vi "Event Handle Loop_Insert.vi"(8 "error in (no error)":errorcluster, 10 "Label":string, 11 "QTab Class in":refnum<class "QTab Class.lvclass">) -> (0 "error out":errorcluster, 3 "QTab Class out":refnum<class "QTab Class.lvclass">)   [LabVIEW 2020, in "QTab.lvlib" / "QTab Class.lvclass"]
uses:
  QTab Class.lvclass
  QTab Class.lvclass/QTab Class.ctl
  QMenu Class/Button Attribute.ctl
  QMenu Class/QMenu Class.lvclass
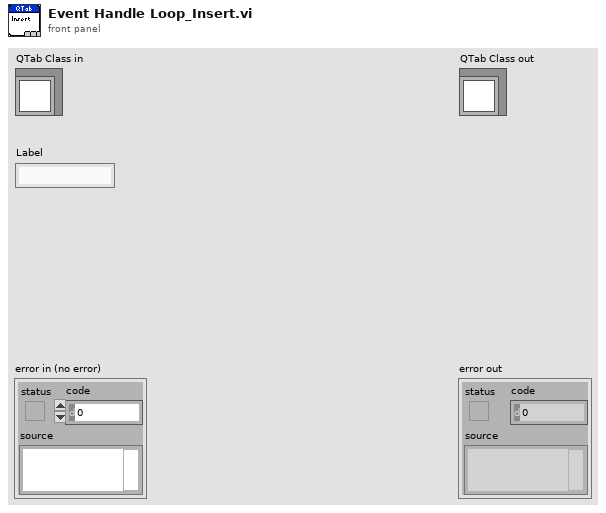
[diagram p1: front panel]
types:
  T1 = typedef "QTab.lvlib/QMenu Class.lvclass/Button Attribute.ctl" = cluster{"Label":string, "Button Text":string, "Closable":bool, "Draggable":bool}
  T2 = typedef "QTab.lvlib/QTab Class.lvclass/Pag Attribute.ctl" = cluster{"VI Refnum":refnum<vi>, "Page Name":string, "Closeable":bool, "Draggable":bool, "Pop-Out":bool}
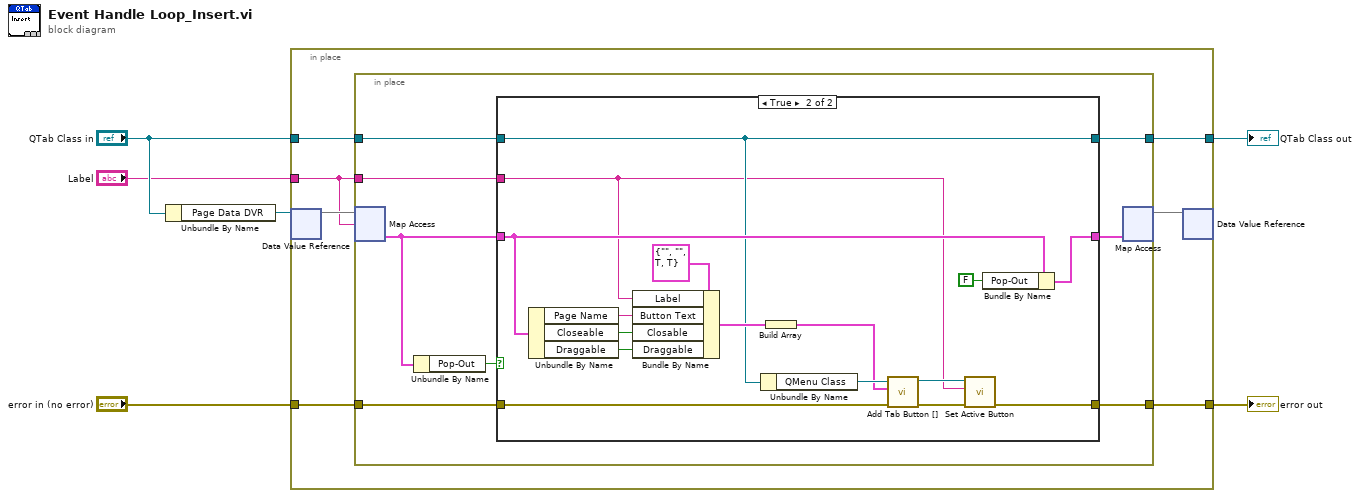
[diagram p0: block diagram]
diagram:
  n1 = Unbundle By Name("QTab Class in") -> ("Page Data DVR"=w5:refnum<data-value>)
  n2 = in-place {
    in-place-border: "error in (no error)" -> [w11]
    in-place-border: "QTab Class in" -> [w12]
    in-place-border: "Label" -> [w7]
    in-place-border: [w10] -> w2
    in-place-border: [w9] -> w1
    n3 = in-place-dvr #1(w5) -> (w13:map{string, T2})  [unwired: 1 out]
    n4 = in-place {
      in-place-border: w12 -> [w19]
      in-place-border: w11 -> [w18]
      in-place-border: [w17] -> w10
      in-place-border: [w16] -> w9
      in-place-border: w7 -> [w14]
      n5 = in-place-map #2(w13, w7) -> (w20:T2)  [unwired: 1 in, 1 out]
      n6 = Unbundle By Name(w20) -> ("Pop-Out"=w21:bool)
      n7 = case shown="True" w21 {
        tunnel: w20 -> [w22 w36]
        tunnel: w19 -> [w23 w29]
        tunnel: w18 -> [w24 w33]
        tunnel: [w23 w29] -> w17
        tunnel: [w24 w26] -> w16
        tunnel: [w22 w34] -> w15
        tunnel: w14 -> [_ w25]
        frame False {
        }
        frame True {
          n8 = Unbundle By Name(w36) -> ("Page Name"=w39:string, "Closeable"=w38:bool, "Draggable"=w37:bool)
          n9 = Bundle By Name(cluster=T1 {"Label"="", "Button Text"="", "Closable"=TRUE, "Draggable"=TRUE} ("Button Attribute"), "Label"=w25, "Button Text"=w39, "Closable"=w38, "Draggable"=w37) -> (w31:T1)
          n10 = Unbundle By Name(w29) -> ("QMenu Class"=w32:refnum<class "QMenu Class.lvclass">)
          n11 = Build Array(w31) -> (w30:T1[])
          n12 = call "Add Tab Button [].vi"("error in (no error)"=w33, "Button Attribute []"=w30, "QMenu Class in"=w32) -> ("error out"=w28:errorcluster, "QMenu Class out"=w27:refnum<class "QMenu Class.lvclass">)  [unwired: 7 in]
          n13 = call "Set Active Button.vi"("error in (no error)"=w28, "Label"=w25, "QMenu Class in"=w27) -> ("error out"=w26:errorcluster)  [unwired: 7 in, 1 out]
          n14 = Bundle By Name(cluster=w36, "Pop-Out"=FALSE) -> (w34:T2)
        }
      }
      n15 = in-place-map #2(w15) -> (w8:map{string, T2})  [unwired: 1 in, 2 out]
    }
    n16 = in-place-dvr #1(w8) -> ()  [unwired: 2 out]
  }
  "error out" <- w1
  "QTab Class out" <- w2
